vi "Music Element To Song.vi"(8 "error in (no error)":errorcluster, 11 "MusicElement":refnum<class "MusicElement.lvclass">) -> (0 "error out":errorcluster, 3 "Song out":refnum<class "Song.lvclass">)   [LabVIEW 2015, in "Song.lvclass"]
uses:
  Song.lvclass
  MusicElement.lvclass
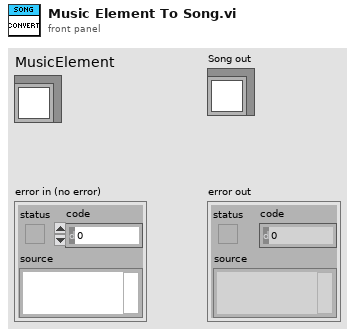
[diagram p1: front panel]
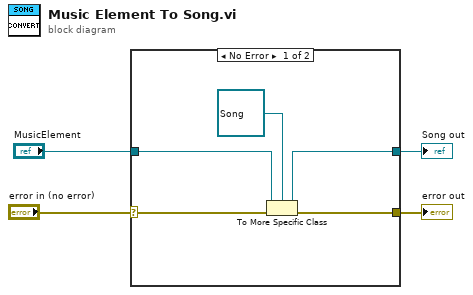
[diagram p0: block diagram]
diagram:
  n1 = case shown="No Error" "error in (no error)" {
    selector: "error in (no error)" -> [w9 w10]
    tunnel: [w7 w10] -> w3
    tunnel: "MusicElement" -> [w8 _]
    tunnel: [w5 _] -> w1
    frame No Error {
      n2 = To More Specific Class(target class=refnum<class "Song.lvclass"> refnum ("Song out"), reference=w8, error in=w9) -> (specific class reference=w5:refnum<class "Song.lvclass">, error out=w7:errorcluster)
    }
    frame Error {
    }
  }
  "error out" <- w3
  "Song out" <- w1
